vi "Set Field.vi"(6 "Positive?":bool, 7 "VISA session":refnum<visa-resource-name>, 8 "error in (no error)":errorcluster, 9 "Desired Field":dbl, 10 "Voltage Limit":dbl=2255.0 format="%.2f", 11 "input cluster":T1) -> (0 "error out":errorcluster, 3 "output cluster":T1, 5 "dup VISA session":refnum<visa-resource-name>)   [LabVIEW 2012]
uses:
  Magna Power Constants.vi
  <vilib>/gmath/NI_Gmath.lvlib
panel:
  out "Current guess":dbl
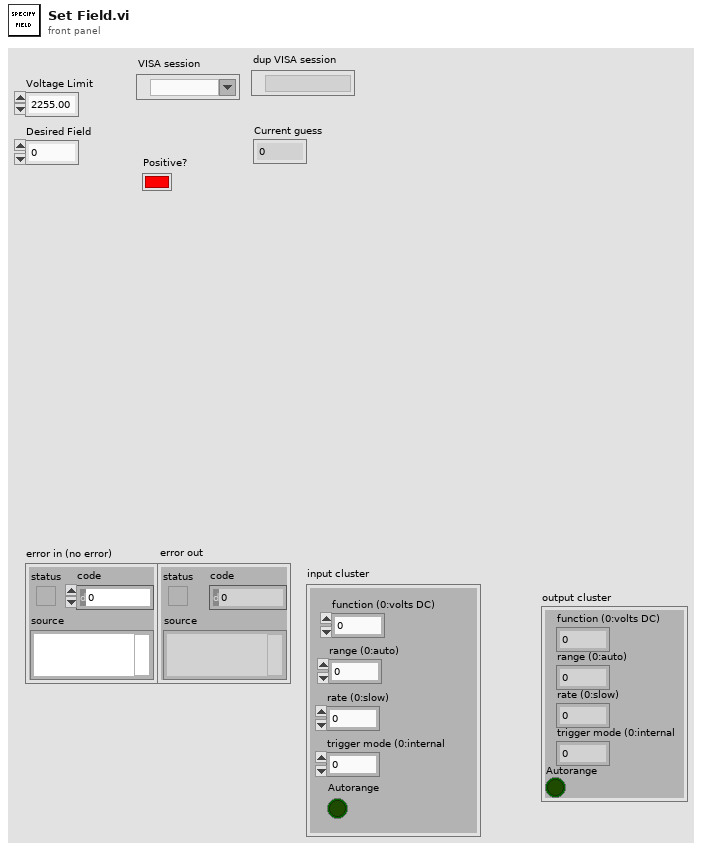
[diagram p1: front panel]
types:
  T1 = cluster{"function (0:volts DC)":i16, "range (0:auto)":i16, "rate (0:slow)":i16, "trigger mode (0:internal":i16, "Autorange":bool}
  T2 = cluster{"Magna Current":dbl[], "Magnetic Field":dbl[], "Fluke Voltage":dbl[]}
  T3 = cluster{"Field":dbl[], "Current Derivative":dbl[]}
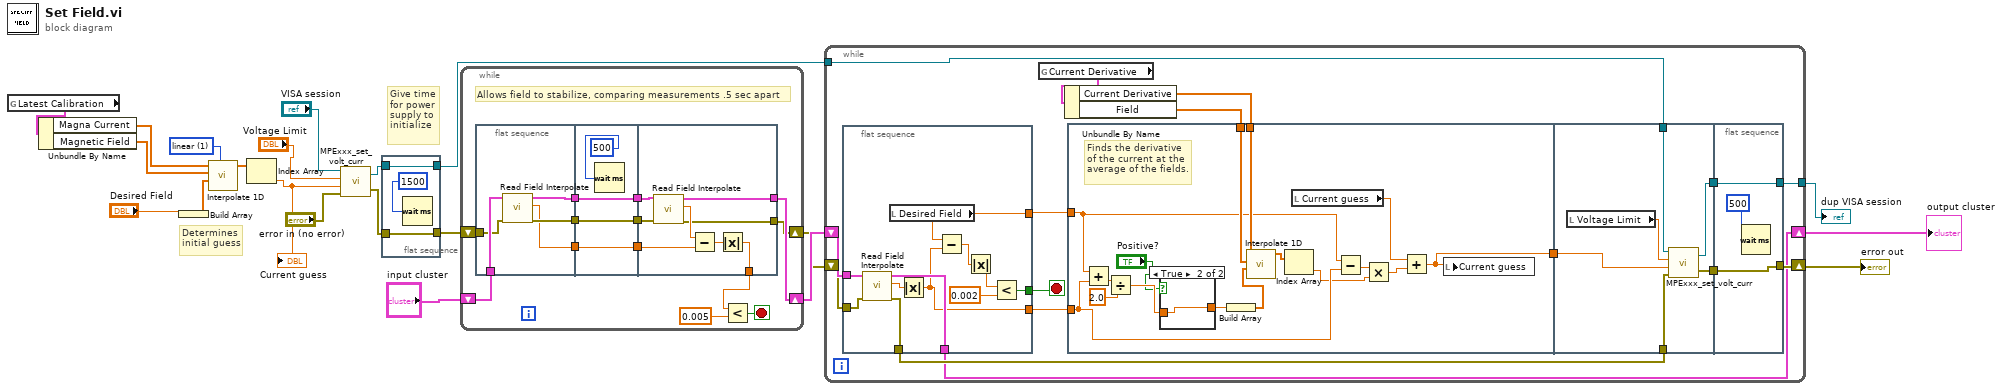
[diagram p0: block diagram]
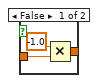
[diagram p2: hidden frame]
diagram:
  w20 = 1 items=["nearest", "linear", "spline", "cubic Hermite", "Lagrange"] ("method")
  # "Give time\nfor power\nsupply to\ninitialize"
  # "Determines\ninitial guess"
  n1 = global read "Magna Power Constants.vi" "Latest Calibration"() -> (w21:T2)
  n2 = Unbundle By Name(w21) -> ("Magna Current"=w12:dbl[], "Magnetic Field"=w13:dbl[])
  n3 = Build Array("Desired Field") -> (w19:dbl[])
  n4 = call <vilib>:"Interpolate 1D.vi"("method"=w20, "xi"=w19, "X"=w13, "Y"=w12) -> ("yi"=w18:dbl[])  [unwired: 5 in, 2 out]
  n5 = Index Array(array=w18) -> (element=w17:dbl)  [unwired: 1 in]
  "Current guess" <- w17
  n6 = call "MPExxx_set_volt_curr.vi"("error in (no error)"="error in (no error)", "Set Current"=w17, "Set Voltage"="Voltage Limit", "VISA session"="VISA session") -> ("error out"=w16:errorcluster, "dup VISA session"=w15:refnum<visa-resource-name>)
  n7 = flat-sequence {
    tunnel: [w23] -> w8
    tunnel: w16 -> [w23]
    tunnel: w15 -> [w22]
    tunnel: [w22] -> w5
    frame #0 {
      n8 = Wait (ms)(milliseconds to wait=u32 1500) -> ()  [unwired: 1 out]
    }
  }
  n9 = while {
    shift-right: [w28] -> w7
    shift-left: "input cluster" -> [w37]
    shift-right: [w26] -> w6
    shift-left: w8 -> [w36]
    stop <- w31 stop-if-true
    # "Allows field to stabilize, comparing measurements .5 sec apart"
    n10 = flat-sequence {
      tunnel: w37 -> [w42]
      tunnel: w36 -> [w41]
      tunnel: [w40] -> w34
      tunnel: [w39] -> w32
      tunnel: [w38] -> w29
      tunnel: [w44] -> w35
      tunnel: w34 -> [w44]
      tunnel: [w45] -> w33
      tunnel: w32 -> [w45]
      tunnel: [w43] -> w30
      tunnel: w29 -> [w43]
      tunnel: w35 -> [w54]
      tunnel: w33 -> [w53]
      tunnel: w30 -> [w50]
      tunnel: [w49] -> w28
      tunnel: [w48] -> w25
      tunnel: [w47] -> w26
      frame #0 {
        n11 = call "Read Field Interpolate.vi"("error in (no error)"=w41, "input cluster"=w42) -> ("error out"=w39:errorcluster, "Field (T)"=w38:dbl, "output cluster"=w40:T1)  [unwired: 7 in]
      }
      frame #1 {
        n12 = Wait (ms)(milliseconds to wait=u32 500) -> ()  [unwired: 1 out]
      }
      frame #2 {
        n13 = call "Read Field Interpolate.vi"("error in (no error)"=w53, "input cluster"=w54) -> ("error out"=w47:errorcluster, "Field (T)"=w51:dbl, "output cluster"=w49:T1)  [unwired: 7 in]
        n14 = Subtract(x=w51, y=w50) -> (x-y=w52:dbl)
        n15 = Absolute Value(x=w52) -> (abs(x)=w48:dbl)
      }
    }
    n16 = Less?(x=w25, y=0.005) -> (x < y?=w31:bool)
  }
  n17 = while {
    tunnel: w5 -> [w62]
    shift-right: [w59] -> w3
    shift-left: w6 -> [w69]
    tunnel: [w57] -> w2
    shift-right: [w55] -> w1
    shift-left: w7 -> [w70]
    stop <- w68 stop-if-true
    n18 = flat-sequence {
      tunnel: w70 -> [w110]
      tunnel: w69 -> [w109]
      tunnel: [w107] -> w68
      tunnel: [w100] -> w64
      tunnel: [w104] -> w63
      tunnel: [w103] -> w61
      tunnel: [w102] -> w55
      frame #0 {
        n19 = call "Read Field Interpolate.vi"("error in (no error)"=w109, "input cluster"=w110) -> ("error out"=w103:errorcluster, "Field (T)"=w101:dbl, "output cluster"=w102:T1)  [unwired: 7 in]
        n20 = local read "Desired Field"() -> (w104:dbl)
        n21 = Absolute Value(x=w101) -> (abs(x)=w100:dbl)
        n22 = Subtract(x=w104, y=w100) -> (x-y=w106:dbl)
        n23 = Absolute Value(x=w106) -> (abs(x)=w105:dbl)
        n24 = Less?(x=w105, y=0.002) -> (x < y?=w107:bool)
      }
    }
    n25 = global read "Magna Power Constants.vi" "Current Derivative"() -> (w65:T3)
    n26 = Unbundle By Name(w65) -> ("Current Derivative"=w66:dbl[], "Field"=w67:dbl[])
    n27 = flat-sequence {
      tunnel: w67 -> [w84]
      tunnel: w66 -> [w83]
      tunnel: w64 -> [w76]
      tunnel: w63 -> [w77]
      tunnel: [w71] -> w60
      tunnel: w62 -> [w96]
      tunnel: w61 -> [w95]
      tunnel: w60 -> [w93]
      tunnel: [w92] -> w58
      tunnel: [w91] -> w56
      tunnel: [w98] -> w59
      tunnel: w58 -> [w98]
      tunnel: [w97] -> w57
      tunnel: w56 -> [w97]
      frame #0 {
        # "Finds the derivative\nof the current at the\naverage of the fields."
        n28 = Add(x=w77, y=w76) -> (x+y=w81:dbl)
        n29 = Divide(x=w81, y=2.0) -> (x/y=w79:dbl)
        n30 = case shown="True" "Positive?" {
          tunnel: w79 -> [w88 w90]
          tunnel: [w87 w90] -> w86
          frame False {
            n31 = Multiply(x=-1.0, y=w88) -> (x*y=w87:dbl)
          }
          frame True {
          }
        }
        n32 = Build Array(w86) -> (w85:dbl[])
        n33 = call <vilib>:"Interpolate 1D.vi"("xi"=w85, "X"=w84, "Y"=w83) -> ("yi"=w82:dbl[])  [unwired: 6 in, 2 out]
        n34 = Index Array(array=w82) -> (element=w74:dbl)  [unwired: 1 in]
        n35 = local read "Current guess"() -> (w73:dbl)
        n36 = Subtract(x=w77, y=w76) -> (x-y=w75:dbl)
        n37 = Multiply(x=w75, y=w74) -> (x*y=w72:dbl)
        n38 = Add(x=w73, y=w72) -> (x+y=w71:dbl)
        n39 = local write "Current guess"(w71) -> ()
      }
      frame #1 {
        n40 = local read "Voltage Limit"() -> (w94:dbl)
        n41 = call "MPExxx_set_volt_curr.vi"("error in (no error)"=w95, "Set Current"=w93, "Set Voltage"=w94, "VISA session"=w96) -> ("error out"=w92:errorcluster, "dup VISA session"=w91:refnum<visa-resource-name>)
      }
      frame #2 {
        n42 = Wait (ms)(milliseconds to wait=u32 500) -> ()  [unwired: 1 out]
      }
    }
  }
  "error out" <- w3
  "output cluster" <- w1
  "dup VISA session" <- w2
